vi "SetVoltageCurrent.vi"(8 "error in (no error)":errorcluster) -> (0 "error out":errorcluster, 1 "CURRENT":dbl, 2 "VOLT":dbl, 3 "COM":string)   [LabVIEW 2020, in "GPP.lvlib"]
uses:
  GPP.lvlib
  <vilib>/Utility/config.llb/Read Key (String).vi
  <vilib>/Utility/config.llb/Read Key (Double).vi
  <vilib>/Utility/config.llb/NI_LVConfig.lvlib
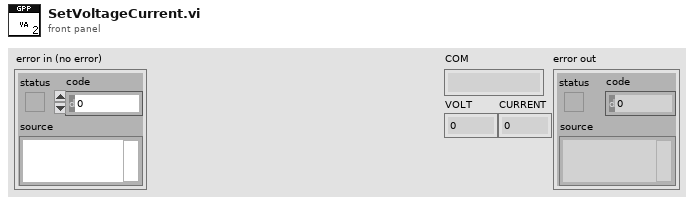
[diagram p1: front panel]
types:
  T1 = typedef "NI_LVConfig.lvlib/Config Data RefNum.ctl" = refnum<k1>
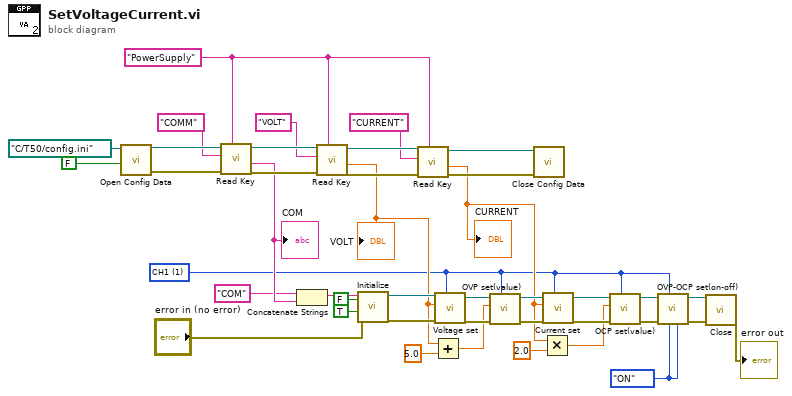
[diagram p0: block diagram]
diagram:
  w1 = enum16{"ON", "OFF"}."ON" ("OVP")
  w4 = u16 1 items=["CH1"=1, "CH2"=2, "CH3"=3, "CH4"=4] ("Channel  (1: CH1)")
  w27 = "PowerSupply" ("section")
  n1 = call <vilib>:"Open Config Data.vi"("create file if necessary (T)"=FALSE, "configuration file path"=path "C:/T50/config.ini") -> ("error out"=w40:errorcluster, "refnum"=w39:T1)  [unwired: 7 in, 1 out]
  n2 = call-poly <vilib>:"Read Key.vi"("section"=w27, "error in (no error)"=w40, "key"="COMM", "refnum"=w39) -> ("error out"=w36:errorcluster, "value"=w33:string, "refnum out"=w35:T1)  [unwired: 4 in, 1 out]
  "COM" <- w33
  n3 = Concatenate Strings("COM" ("string"), w33) -> (w25:string)
  n4 = call-poly <vilib>:"Read Key.vi"("section"=w27, "error in (no error)"=w36, "key"="VOLT", "refnum"=w35) -> ("error out"=w31:errorcluster, "value"=w14:dbl, "refnum out"=w30:T1)  [unwired: 4 in, 1 out]
  "VOLT" <- w14
  n5 = call "Initialize.vi"("error in (no error)"="error in (no error)", "Reset (True)"=TRUE, "ID Query (True)"=FALSE, "VISA resource name"=w25) -> ("error out"=w22:errorcluster, "VISA resource name out"=w21:refnum<visa-resource-name>)  [unwired: 5 in, 1 out]
  n6 = call-poly <vilib>:"Read Key.vi"("section"=w27, "error in (no error)"=w31, "key"="CURRENT", "refnum"=w30) -> ("error out"=w28:errorcluster, "value"=w9:dbl, "refnum out"=w29:T1)  [unwired: 4 in, 1 out]
  "CURRENT" <- w9
  n7 = Add(x=w14, y=5.0) -> (x+y=w12:dbl)
  n8 = call "Voltage set.vi"("Channel  (1: CH1)"=w4, "error in (no error)"=w22, "Voltage"=w14, "VISA resource name"=w21) -> ("error out"=w18:errorcluster, "VISA resource name out"=w17:refnum<visa-resource-name>)  [unwired: 6 in]
  n9 = call "OVP set(value).vi"("Channel  (1: CH1)"=w4, "error in (no error)"=w18, "OVP"=w12, "VISA resource name"=w17) -> ("error out"=w15:errorcluster, "VISA resource name out"=w16:refnum<visa-resource-name>)  [unwired: 6 in]
  n10 = call <vilib>:"Close Config Data.vi"("error in (no error)"=w28, "refnum"=w29) -> ()  [unwired: 8 in, 2 out]
  n11 = Multiply(x=w9, y=2.0) -> (x*y=w7:dbl)
  n12 = call "Current set.vi"("Channel  (1: CH1)"=w4, "error in (no error)"=w15, "Current"=w9, "VISA resource name"=w16) -> ("error out"=w11:errorcluster, "VISA resource name out"=w10:refnum<visa-resource-name>)  [unwired: 6 in]
  n13 = call "OCP set(value).vi"("Channel  (1: CH1)"=w4, "error in (no error)"=w11, "OCP"=w7, "VISA resource name"=w10) -> ("error out"=w6:errorcluster, "VISA resource name out"=w5:refnum<visa-resource-name>)  [unwired: 6 in]
  n14 = call "OVP-OCP set(on-off).vi"("OCP"=w1, "OVP"=w1, "Channel  (1: CH1)"=w4, "error in (no error)"=w6, "VISA resource in"=w5) -> ("error out"=w2:errorcluster, "VISA resource name out"=w3:refnum<visa-resource-name>)  [unwired: 5 in]
  n15 = call "Close.vi"("error in (no error)"=w2, "VISA resource name"=w3) -> ("error out"=→"error out":errorcluster)  [unwired: 9 in]
